vi "UMLEditor CreateAggregationAttributes.vi"(2 "ClassAggregation":refnum<class "AbstractEdge.lvclass">, 5 "error in (no error)":errorcluster) -> (15 "NodeModified":refnum<class "AbstractNode.lvclass">, 16 "Modified?":bool, 19 "error out":errorcluster)   [LabVIEW 2012]
doc: "Gets current diagram values"
uses:
  <resource>/Framework/Providers/Open_GDS/UML/AbstractEdge_class/AbstractEdge.lvclass
  <resource>/Framework/Providers/Open_GDS/UML/AbstractNode_class/AbstractNode.lvclass
  <resource>/Framework/Providers/Open_GDS/UML/ClassNode_class/ExternalSetTypes.ctl
  <resource>/Framework/Providers/Open_GDS/UML/ClassNode_class/ClassNode.lvclass
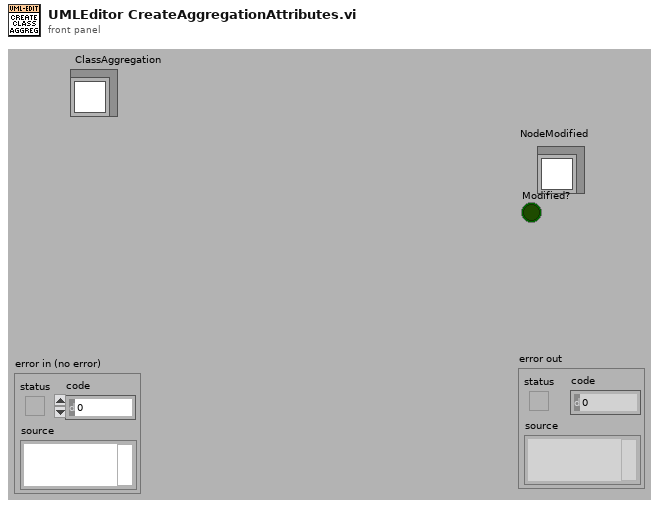
[diagram p1: front panel]
types:
  T1 = typedef "ClassNode.lvclass/ExternalSetTypes.ctl" = enum16{"Name", "Attributes", "Methods", "Position", "ShowMethods", "ShowAttributes", "ClassPath"}
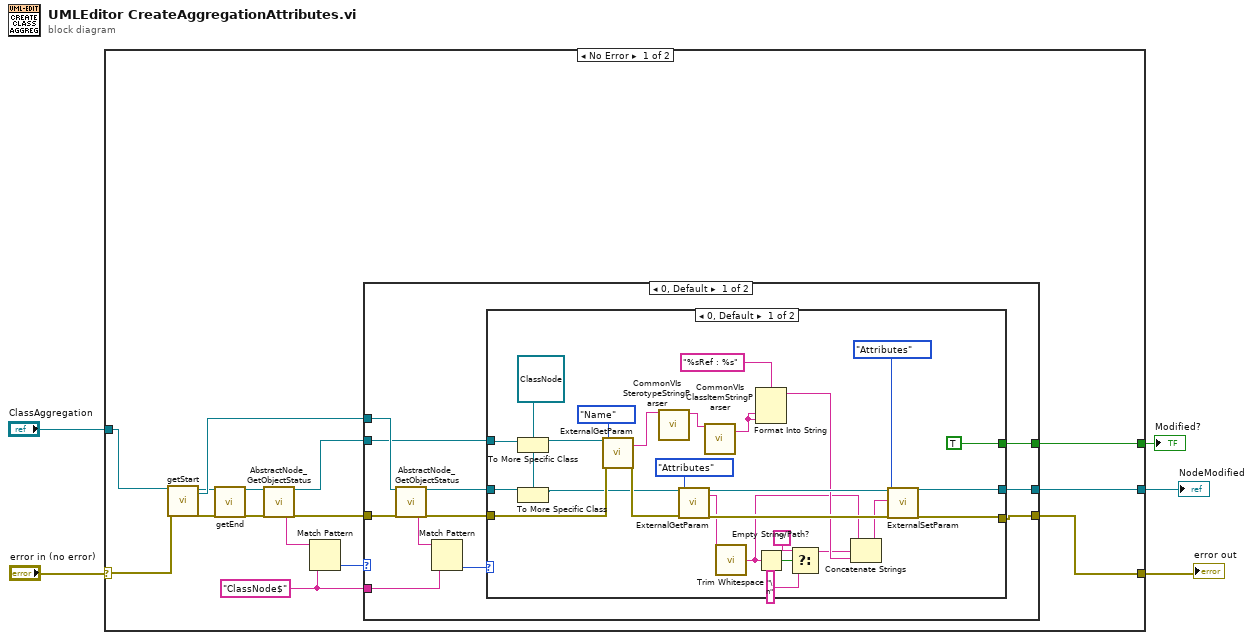
[diagram p0: block diagram]
diagram:
  n1 = case shown="No Error" "error in (no error)" {
    selector: "error in (no error)" -> [w20 w61]
    tunnel: [w9 w61] -> w4
    tunnel: "ClassAggregation" -> [w19 _]
    tunnel: [w7 _] -> w2
    tunnel: [w6 _] -> w1
    frame No Error {
      w12 = "ClassNode$" ("regular expression")
      n2 = call-dynamic "getStart.vi"("reference"=w19, "error in (no error)"=w20) -> ("reference out"=w17:refnum<class "AbstractEdge.lvclass">, "startNode"=w18:refnum<class "AbstractNode.lvclass">, "error out"=w16:errorcluster)  [unwired: 14 in, 1 out]
      n3 = call-dynamic "getEnd.vi"("reference"=w17, "error in (no error)"=w16) -> ("endNode"=w15:refnum<class "AbstractNode.lvclass">, "error out"=w14:errorcluster)  [unwired: 14 in, 2 out]
      n4 = call <resource>:"AbstractNode_GetObjectStatus.vi"("reference in"=w15, "error in (no error)"=w14) -> ("Class name"=w13:string, "reference out"=w8:refnum<class "AbstractNode.lvclass">, "error out"=w10:errorcluster)  [unwired: 15 out]
      n5 = Match Pattern(string=w13, regular expression=w12) -> (offset past match=w11:i32)  [unwired: 4 out]
      n6 = case shown="0, Default" w11 {
        tunnel: w18 -> [w27 _]
        tunnel: w12 -> [w26 _]
        tunnel: w10 -> [w24 w60]
        tunnel: [w25 w60] -> w9
        tunnel: w8 -> [w23 _]
        tunnel: [w22 _] -> w7
        tunnel: [w21 _] -> w6
        frame 0, Default {
          n7 = call <resource>:"AbstractNode_GetObjectStatus.vi"("reference in"=w27, "error in (no error)"=w24) -> ("Class name"=w31:string, "reference out"=w28:refnum<class "AbstractNode.lvclass">, "error out"=w29:errorcluster)  [unwired: 15 out]
          n8 = Match Pattern(string=w31, regular expression=w26) -> (offset past match=w30:i32)  [unwired: 4 out]
          n9 = case shown="0, Default" w30 {
            tunnel: w29 -> [w52 w59]
            tunnel: w28 -> [w34 _]
            tunnel: [w54 w59] -> w25
            tunnel: w23 -> [w36 _]
            tunnel: [w46 _] -> w22
            tunnel: [TRUE _] -> w21
            frame 0, Default {
              w33 = refnum<class "ClassNode.lvclass"> refnum ("reference")
              n10 = To More Specific Class(target class=w33, reference=w36) -> (specific class reference=w35:refnum<class "ClassNode.lvclass">)  [unwired: 1 in, 1 out]
              n11 = To More Specific Class(target class=w33, reference=w34) -> (specific class reference=w32:refnum<class "ClassNode.lvclass">)  [unwired: 1 in, 1 out]
              n12 = call <resource>:"ExternalGetParam.vi"("reference"=w35, "setParameter"=ExternalSetTypes."Name", "error in (no error)"=w52) -> ("string"=w50:string, "error out"=w51:errorcluster)  [unwired: 15 out]
              n13 = call <resource>:"CommonVIs SterotypeStringParser.vi"("SterotypeStringIn"=w50) -> ("Name"=w38:string)  [unwired: 18 out]
              n14 = call <resource>:"ExternalGetParam.vi"("reference"=w32, "setParameter"=ExternalSetTypes."Attributes", "error in (no error)"=w51) -> ("reference out"=w57:refnum<class "ClassNode.lvclass">, "string"=w40:string, "error out"=w56:errorcluster)  [unwired: 14 out]
              n15 = call <resource>:"CommonVIs ClassItemStringParser.vi"("ClassItemNameIn"=w38) -> ("Name"=w37:string)  [unwired: 18 out]
              n16 = call <vilib>:"Trim Whitespace.vi"("string"=w40) -> ("trimmed string"=w39:string)  [unwired: 1 in]
              n17 = Format Into String(format string="%sRef : %s", w37, w37) -> (resulting string=w48:string)  [unwired: 2 in, 1 out]
              n18 = Empty String/Path?(string/path=w39) -> (empty?=w44:bool)
              n19 = Select(t="", s=w44, f="\n") -> (s? t:f=w43:string)
              n20 = Concatenate Strings(w39, w43, w48) -> (w47:string)
              n21 = call-dynamic "ExternalSetParam.vi"("reference"=w57, "setParameter"=ExternalSetTypes."Attributes", "string"=w47, "error in (no error)"=w56) -> ("reference out"=w46:refnum<class "ClassNode.lvclass">, "error out"=w54:errorcluster)  [unwired: 14 in]
            }
            frame -1 {
            }
          }
        }
        frame -1 {
        }
      }
    }
    frame Error {
    }
  }
  "error out" <- w4
  "NodeModified" <- w2
  "Modified?" <- w1
